vi "SerialReadFromArduino.vi"() -> ()   [LabVIEW 2020]
uses:
  <vilib>/Instr/_visa.llb/VISA Configure Serial Port (Instr).vi
panel:
  out "Waveform Chart":dbl(graph)
  in  "stop":bool
  out "read buffer":string
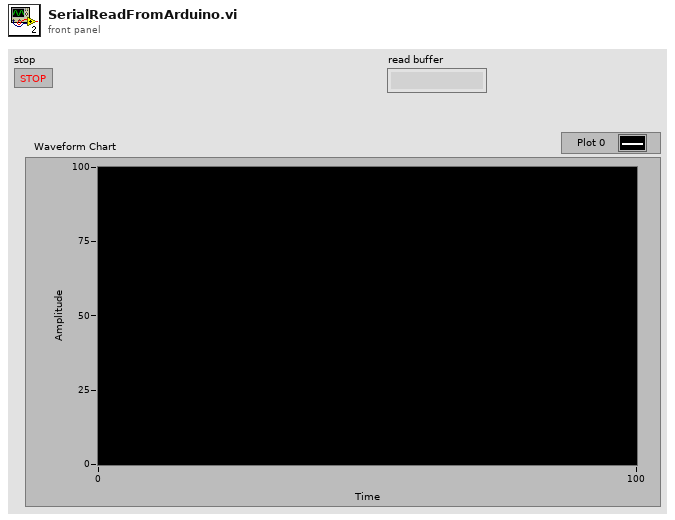
[diagram p1: front panel]
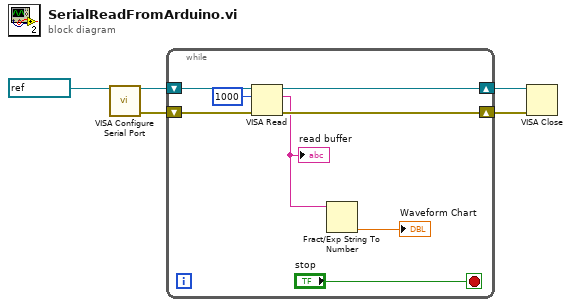
[diagram p0: block diagram]
diagram:
  n1 = call-poly "VISA Configure Serial Port"("VISA resource name"=refnum<visa-resource-name> "COM4") -> ("VISA resource name out"=w5:refnum<visa-resource-name>, "error out"=w4:errorcluster)  [unwired: 9 in, 4 out]
  n2 = while {
    shift-right: [w11] -> w3
    shift-left: w5 -> [w13]
    shift-right: [w10] -> w2
    shift-left: w4 -> [w12]
    stop <- "stop" stop-if-true
    n3 = VISA Read(VISA resource name=w13, byte count=u32 1000, error in (no error)=w12) -> (VISA resource name out=w11:refnum<visa-resource-name>, read buffer=w6:string, error out=w10:errorcluster)  [unwired: 1 out]
    "read buffer" <- w6
    n4 = Fract/Exp String To Number(string=w6) -> (number=→"Waveform Chart":dbl)  [unwired: 3 in, 1 out]
  }
  n5 = VISA Close(VISA resource name=w3, error in (no error)=w2) -> ()  [unwired: 1 out]
